vi "HW_GEN - Read Module Channel Configurations(bin).vi"(8 "error in":errorcluster caption="错误输入", 11 "ModuCFG path":path) -> (0 "error out":errorcluster caption="错误输出", 3 "ModCFG out":T1[](array[typedef]))   [LabVIEW 2016]
uses:
  Ctrls/HardWare _ Module Configuration.ctl
panel:
  # "ModTag:\nModName>>ModSN>>ChanType"
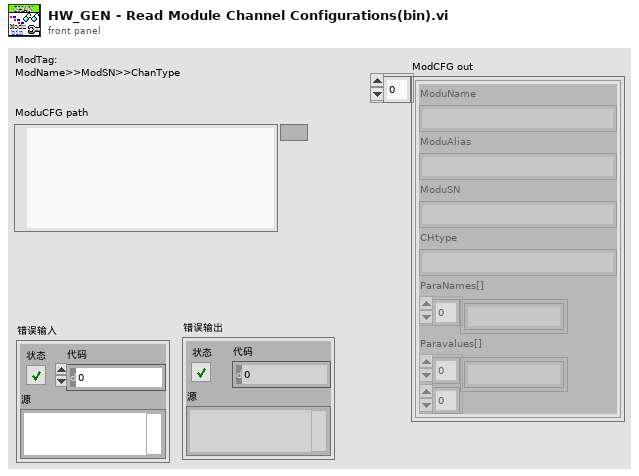
[diagram p1: front panel]
types:
  T1 = typedef "HardWare _ Module Configuration.ctl" = cluster{"ModuName":string, "ModuAlias":string, "ModuSN":string, "CHtype":string, "ParaNames[]":string[], "Paravalues[]":string[][]}
  T2 = enum16{"open", "replace", "create", "open or create", "replace or create", "replace or create with confirmation"}
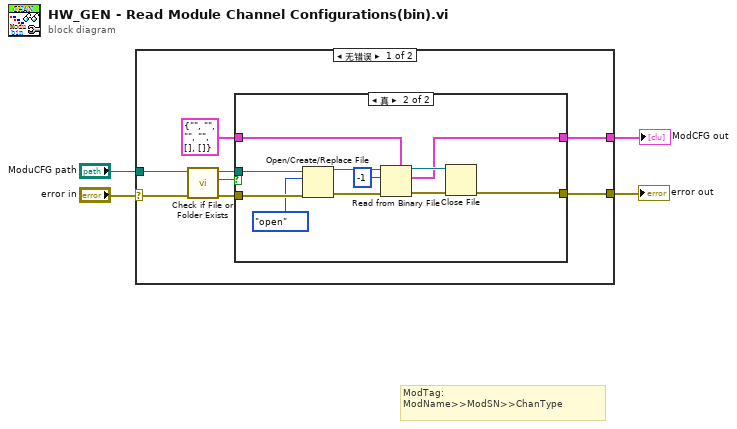
[diagram p0: block diagram]
diagram:
  # "ModTag:\nModName>>ModSN>>ChanType"
  n1 = case shown="无错误" "error in" {
    selector: "error in" -> [w11 w25]
    tunnel: [w7 w25] -> w4
    tunnel: "ModuCFG path" -> [w12 _]
    tunnel: [w5 _] -> w1
    frame No Error {
      n2 = call <vilib>:"Check if File or Folder Exists.vi"("error in (no error)"=w11, "path"=w12) -> ("error out"=w10:errorcluster, "file or folder exists?"=w9:bool, "dup path"=w8:path)  [unwired: 7 in]
      n3 = case shown="真" w9 {
        tunnel: [w13 w24] -> w7
        tunnel: w10 -> [w13 w23]
        tunnel: w8 -> [_ w22]
        tunnel: T1 {"ModuName"="", "ModuAlias"="", "ModuSN"="", "CHtype"="", "ParaNames[]"=[], "Paravalues[]"=[]} ("ModuCfg") -> [_ w21]
        tunnel: [_ w14] -> w5
        frame False {
          # "文件不存在，则新建"
        }
        frame True {
          n4 = Open/Create/Replace File(file path (use dialog)=w22, error in=w23, operation (0:open)=T2."open") -> (refnum out=w18:refnum<file>, error out=w19:errorcluster)  [unwired: 3 in, 1 out]
          n5 = Read from Binary File(5:w21, 8:w19, 10:-1 ("count (1)"), 11:w18) -> (0:w16:errorcluster, 2:w14:T1[], 3:w15:refnum<file>)  [unwired: 2 in, 1 out]
          n6 = Close File(refnum=w15, error in=w16) -> (error out=w24:errorcluster)  [unwired: 1 out]
        }
      }
    }
    frame Error {
    }
  }
  "error out" <- w4
  "ModCFG out" <- w1
